vi "LossyEnqueueMessage.vi"(8 "error in":errorcluster, 10 "Message":refnum<class "Message.lvclass">, 11 "PrefixQueue in":refnum<class "PrefixQueue.lvclass">) -> (0 "error out":errorcluster, 1 "Overflow?":bool, 2 "Overflow Message":refnum<class "Message.lvclass">, 3 "PrefixQueue out":refnum<class "PrefixQueue.lvclass">)   [LabVIEW 2017, in "LapDog.Messaging.v3.PrefixQueue.lvlib" / "PrefixQueue.lvclass"]
doc: "Adds an element to the queue. If the queue is full, the first element is removed from the queue and discarded.\n\nThis method executes regardless of the error in state."
uses:
  PrefixQueue.lvclass
  LapDog.Messaging/Message/Message.lvclass
  PrefixQueue.lvclass/PrefixQueue.ctl
  LapDog.Messaging/MessageQueue/MessageQueue.lvclass
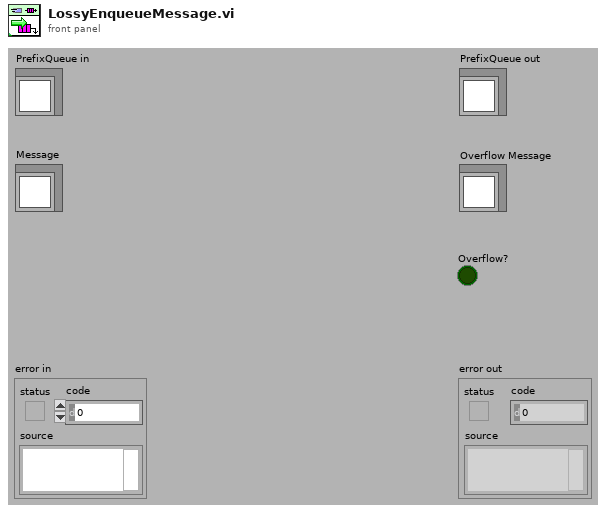
[diagram p1: front panel]
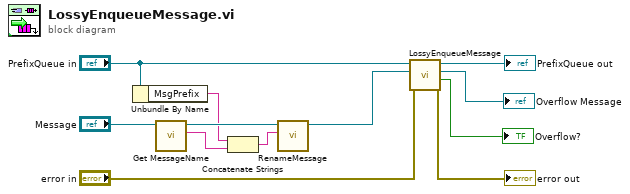
[diagram p0: block diagram]
diagram:
  n1 = Unbundle By Name("PrefixQueue in") -> ("MsgPrefix"=w3:string)
  n2 = call "Get MessageName.vi"("Message in"="Message") -> ("Message Name"=w6:string, "Message out"=w8:refnum<class "Message.lvclass">)  [unwired: 8 in, 1 out]
  n3 = Concatenate Strings(w3, w6) -> (w7:string)
  n4 = call "RenameMessage.vi"("Message Name"=w7, "Message in"=w8) -> ("Message out"=w4:refnum<class "Message.lvclass">)  [unwired: 8 in, 1 out]
  n5 = call-parent "LossyEnqueueMessage.vi"("error in"="error in", "Message"=w4, "MessageQueue in"="PrefixQueue in") -> ("error out"=→"error out":errorcluster, "Overflow?"=→"Overflow?":bool, "Overflow Message"=→"Overflow Message":refnum<class "Message.lvclass">, "MessageQueue out"=→"PrefixQueue out":refnum<class "PrefixQueue.lvclass">)  [unwired: 5 in]
